vi "Enqueue Single Message.vi"(8 "error in (no error)":errorcluster, 10 "queue in":refnum<queue>, 11 "Message in":refnum<class "Message.lvclass">) -> (0 "error out":errorcluster, 2 "queue out":refnum<queue>)   [LabVIEW 2021, in "Architecture.lvlib" / "Message.lvclass"]
doc: "Enqueue a message in a message local queue"
uses:
  Message.lvclass
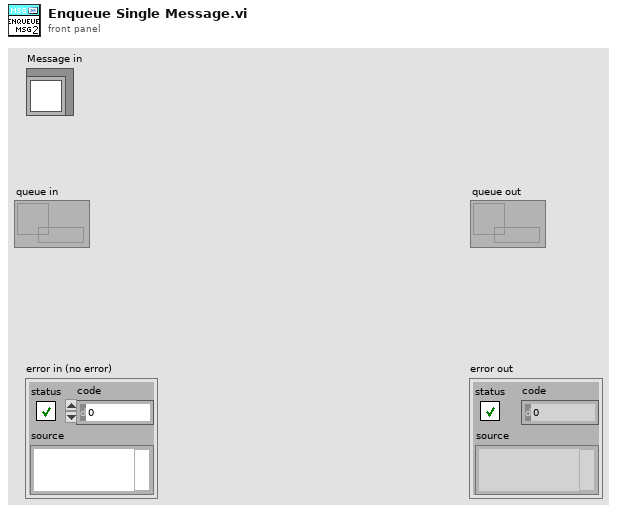
[diagram p1: front panel]
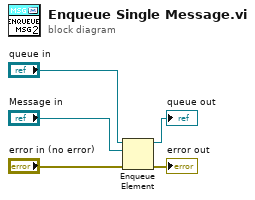
[diagram p0: block diagram]
diagram:
  n1 = Enqueue Element(queue="queue in", element="Message in", error in (no error)="error in (no error)") -> (queue out=→"queue out":refnum<queue>, error out=→"error out":errorcluster)  [unwired: 1 in, 1 out]
